vi "Delete Annotation.vi"(8 "error in (no error)":errorcluster, 10 "Name":string, 11 "FSM in":refnum<class "FSM.Graph.lvclass">) -> (0 "error out":errorcluster, 2 "Changed?":bool, 3 "FSM out":refnum<class "FSM.Graph.lvclass">)   [LabVIEW 2015, in "FSM.Graph.lvclass"]
uses:
  FSM.Graph.lvclass
  FSM.Edge/FSM.Edge.lvclass
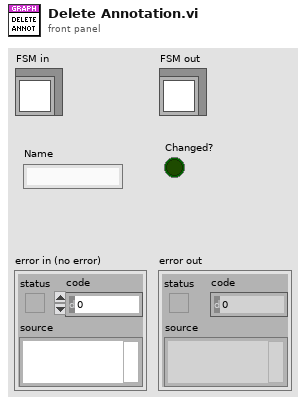
[diagram p1: front panel]
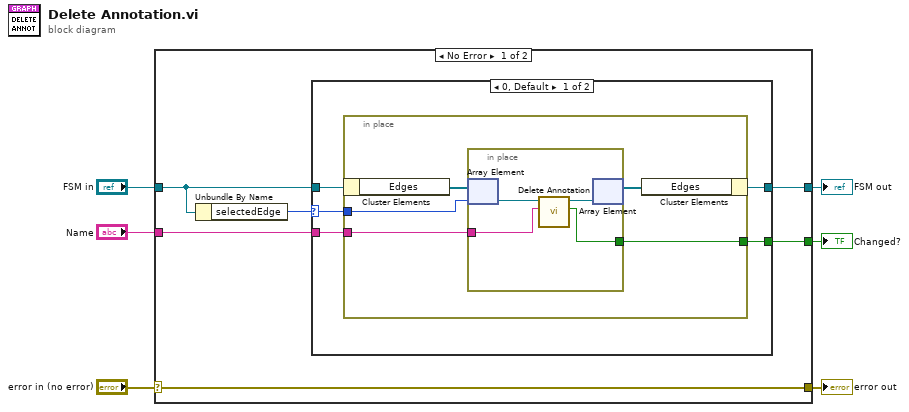
[diagram p0: block diagram]
diagram:
  n1 = case shown="No Error" "error in (no error)" {
    selector: "error in (no error)" -> [w12 w29]
    tunnel: [w12 w29] -> w5
    tunnel: [w9 w28] -> w3
    tunnel: "FSM in" -> [w10 w28]
    tunnel: "Name" -> [w8 _]
    tunnel: [w7 _] -> w1
    frame No Error {
      n2 = Unbundle By Name(w10) -> ("selectedEdge"=w11:i32)
      n3 = case shown="0, Default" w11 {
        selector: w11 -> [w16 _]
        tunnel: w10 -> [w17 w27]
        tunnel: [w14 w27] -> w9
        tunnel: w8 -> [w15 _]
        tunnel: [w13 _] -> w7
        frame 0, Default {
          n4 = in-place {
            in-place-border: w16 -> [w21]
            in-place-border: w15 -> [w20]
            in-place-border: [w18] -> w13
            n5 = in-place-cluster #1(w17) -> ("Edges"=w22:refnum<class "FSM.Edge.lvclass">[])
            n6 = in-place {
              in-place-border: w20 -> [w24]
              in-place-border: [w23] -> w18
              n7 = in-place-array #2(w22, w21) -> (w26:refnum<class "FSM.Edge.lvclass">)
              n8 = call "Delete Annotation.vi"("Name"=w24, "FSM.Edge in"=w26) -> ("Changed?"=w23:bool, "FSM.Edge out"=w25:refnum<class "FSM.Edge.lvclass">)  [unwired: 7 in, 1 out]
              n9 = in-place-array #2(w25) -> (w19:refnum<class "FSM.Edge.lvclass">[])  [unwired: 1 out]
            }
            n10 = in-place-cluster #1("Edges"=w19) -> (w14:refnum<class "FSM.Graph.lvclass">)
          }
        }
        frame -1 {
        }
      }
    }
    frame Error {
    }
  }
  "error out" <- w5
  "FSM out" <- w3
  "Changed?" <- w1
